vi "scan_v24.vi"(8 "error in (no error)":errorcluster, 11 "Input":string="34,45,89") -> (0 "error out":errorcluster, 3 "Output":string)   [LabVIEW 2014]
uses:
  <userlib>/Nanonis Prog Interface V5/Nanonis Prog Interface.lvlib
panel:
  in  "Channel":u8(ring)=14 items=["Current"=0, "Z (m)"=14]
  in  "Direction: Fwd/Bwd (T=Fwd)":bool=TRUE
  in  "milliseconds to wait":u32=3000
  in  "Angle (deg)":sgl=nan caption="Angle (deg) (NaN=no change)" format="%.2f"
  in  "Size (m)":cluster{"Width":sgl, "Height":sgl}={"Width"=1e-08, "Height"=1e-08} caption="Size (m) (NaN=no change)" {"Height" format="%.2p"; "Width" format="%.2p"}
  out "size(s)":i32=3
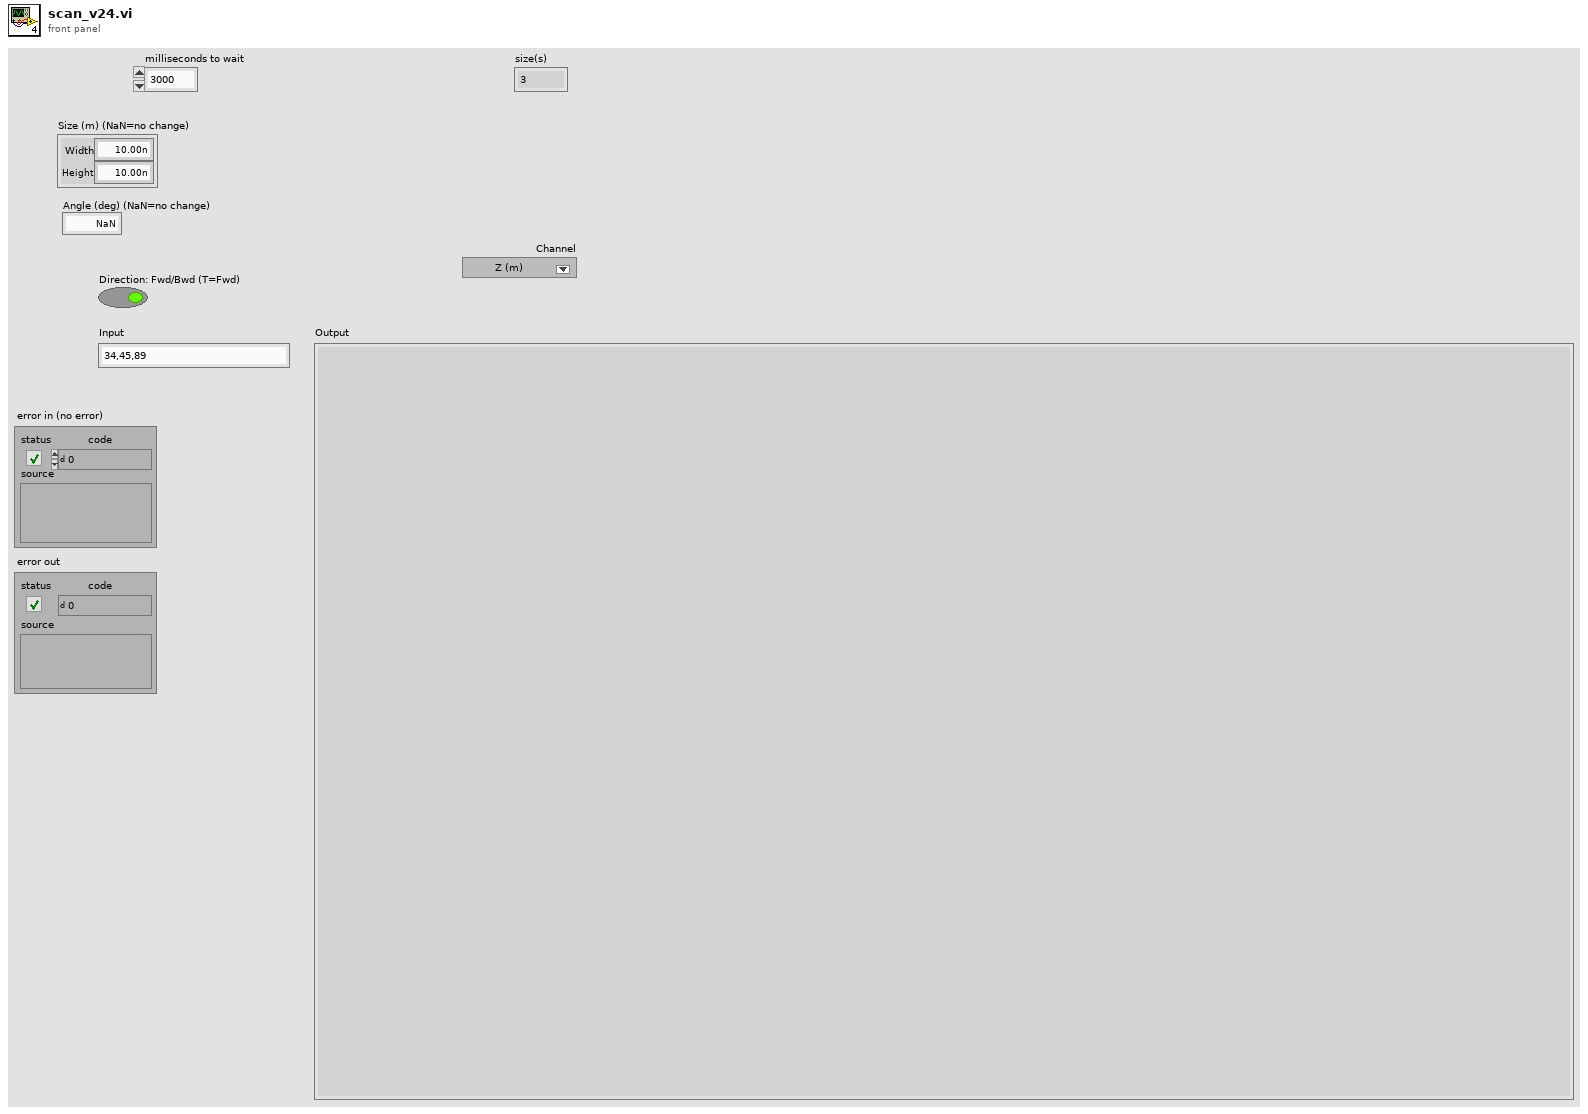
[diagram p1: front panel]
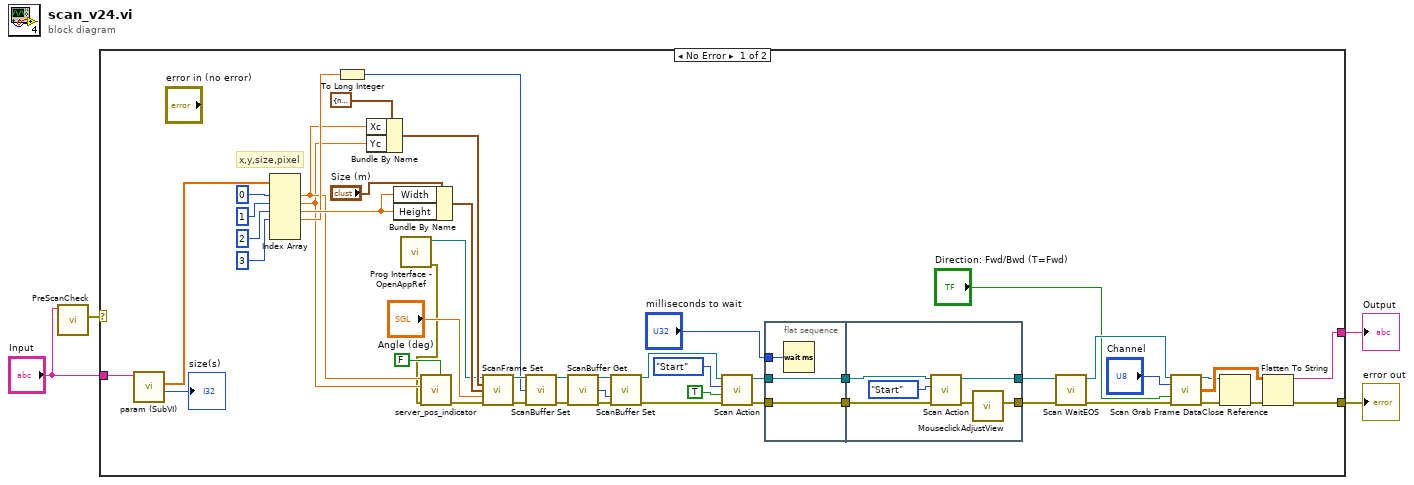
[diagram p0: block diagram]
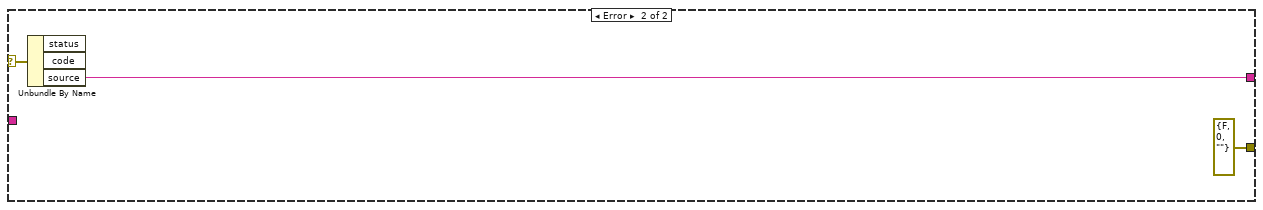
[diagram p2: hidden frame]
diagram:
  n1 = call "PreScanCheck.vi"("Input"="Input") -> ("error"=w1:errorcluster)  [unwired: 8 in, 2 out]
  n2 = case shown="No Error" w1 {
    selector: w1 -> [_ w64]
    tunnel: [w25 w63] -> w4
    tunnel: [w13 errorcluster {"status"=FALSE, "code"=0, "source"=""} ("error out")] -> w3
    tunnel: "Input" -> [w5 _]
    frame No Error {
      # "x,y,size,pixel"
      n3 = call <userlib>:"param (SubVI).vi"("Input"=w5) -> ("num"=→"size(s)":i32, "parm"=w50:dbl[])  [unwired: 8 in, 1 out]
      n4 = Index Array(array=w50, index #1=0 ("index"), index #2=1 ("index"), index #3=2 ("index"), index #4=3 ("index")) -> (element #1=w11:dbl, element #2=w10:dbl, element #3=w29:dbl, element #4=w27:dbl)  [unwired: 2 in, 2 out]
      n5 = To Long Integer(number=w27) -> (32bit integer=w26:i32)
      n6 = Bundle By Name(cluster=cluster{"Xc":sgl, "Yc":sgl} {"Xc"=nan, "Yc"=nan} ("Center coordinates (m)"), "Xc"=w11, "Yc"=w10) -> (w48:cluster{"Xc":sgl, "Yc":sgl})
      n7 = Bundle By Name(cluster="Size (m)", "Width"=w29, "Height"=w29) -> (w28:cluster{"Width":sgl, "Height":sgl})
      n8 = call <userlib>:"Prog Interface - OpenAppRef.vi"() -> ("Error out"=w7:errorcluster, "Application reference"=w6:refnum<vi>)  [unwired: 6 in]
      n9 = call "server_pos_indicator.vi"("reset"=FALSE, "error in"=w7, "yc"=w10, "xc"=w11) -> ("error out"=w8:errorcluster)  [unwired: 7 in]
      n10 = call <userlib>:"ScanFrame Set.vi"("Application ref in"=w6, "Center coordinates (m)"=w48, "Size (m)"=w28, "Angle (deg)"="Angle (deg)", "error in (no error)"=w8) -> ("Application ref out"=w46:refnum<vi>, "error out"=w45:errorcluster)  [unwired: 9 in]
      n11 = call <userlib>:"ScanBuffer Set.vi"("Application ref in"=w46, "Pixels"=w26, "error in (no error)"=w45) -> ("Application ref out"=w19:refnum<vi>, "error out"=w18:errorcluster)  [unwired: 11 in]
      n12 = call <userlib>:"ScanBuffer Get.vi"("Application ref in"=w19, "error in (no error)"=w18) -> ("Application ref out"=w21:refnum<vi>, "Pixels/line"=w22:i32, "error out"=w20:errorcluster)  [unwired: 9 in, 2 out]
      n13 = call <userlib>:"ScanBuffer Set.vi"("Application ref in"=w21, "Lines"=w22, "error in (no error)"=w20) -> ("Application ref out"=w17:refnum<vi>, "error out"=w16:errorcluster)  [unwired: 11 in]
      n14 = call <userlib>:"Scan Action.vi"("error in (no error)"=w16, "Direction: up/down (T=up)"=TRUE, "Scan action (Start)"=enum16{"Start", "Stop", "Pause", "Resume"}."Start", "Application ref in"=w17) -> ("error out"=w41:errorcluster, "Application ref out"=w42:refnum<vi>)  [unwired: 5 in]
      n15 = flat-sequence {
        tunnel: w42 -> [w55]
        tunnel: w41 -> [w54]
        tunnel: "milliseconds to wait" -> [w56]
        tunnel: [w55] -> w53
        tunnel: [w54] -> w52
        tunnel: w53 -> [w62]
        tunnel: w52 -> [w61]
        tunnel: [w59] -> w39
        tunnel: [w57] -> w38
        frame #0 {
          n16 = Wait (ms)(milliseconds to wait=w56) -> ()  [unwired: 1 out]
        }
        frame #1 {
          n17 = call <userlib>:"Scan Action.vi"("error in (no error)"=w61, "Scan action (Start)"=enum16{"Start", "Stop", "Pause", "Resume"}."Start", "Application ref in"=w62) -> ("error out"=w58:errorcluster, "Application ref out"=w59:refnum<vi>)  [unwired: 6 in]
          n18 = call "MouseclickAdjustView.vi"("error in (no error)"=w58) -> ("error out"=w57:errorcluster)  [unwired: 10 in]
        }
      }
      n19 = call <userlib>:"Scan WaitEOS.vi"("error in (no error)"=w38, "Application ref in"=w39) -> ("error out"=w35:errorcluster, "Application ref out"=w37:refnum<vi>)  [unwired: 5 in, 2 out]
      n20 = call <userlib>:"Scan Grab Frame Data.vi"("Application ref in"=w37, "Channel index (0-23)"="Channel", "Direction: Fwd/Bwd (T=Fwd)"="Direction: Fwd/Bwd (T=Fwd)", "error in (no error)"=w35) -> ("Application ref out"=w15:refnum<vi>, "Scan frame data"=w23:sgl[][], "error out"=w14:errorcluster)  [unwired: 7 in, 2 out]
      n21 = Close Reference(reference=w15, error in (no error)=w14) -> (error out=w9:errorcluster)
      n22 = Flatten To String(anything=w23, error in (no error)=w9) -> (data string=w25:string, error out=w13:errorcluster)  [unwired: 2 in, 1 out]
    }
    frame Error {
      n23 = Unbundle By Name(w64) -> ("source"=w63:string)  [unwired: 2 out]
    }
  }
  "Output" <- w4
  "error out" <- w3
